vi "Accel Interpret.vi"(1 "LSB":u8, 2 "MSB":u8) -> (0 "Value":i16)   [LabVIEW 2010]
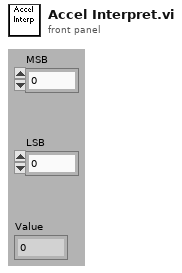
[diagram p1: front panel]
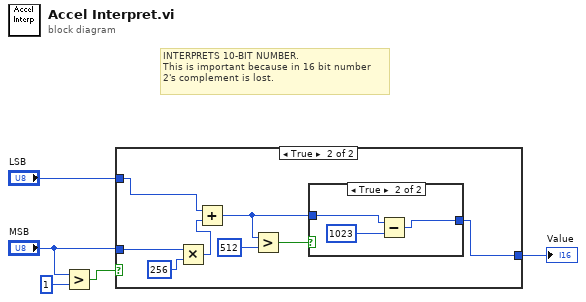
[diagram p0: block diagram]
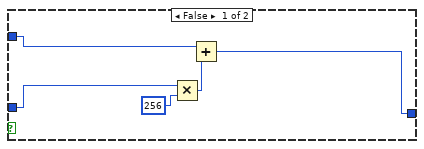
[diagram p2: hidden frame]
diagram:
  # "INTERPRETS 10-BIT NUMBER.\nThis is important because in 16 bit number\n2's complement is lost."
  n1 = Greater?(x="MSB", y=i16 1) -> (0:w4:bool)
  n2 = case shown="True" w4 {
    tunnel: "MSB" -> [w7 w13]
    tunnel: "LSB" -> [w8 w14]
    tunnel: [w6 w15] -> w5
    frame False {
      n3 = Multiply(x=w7, y=u16 256) -> (x*y=w9:u16)
      n4 = Add(x=w8, y=w9) -> (x+y=w6:u16)
    }
    frame True {
      n5 = Multiply(x=w13, y=i16 256) -> (x*y=w12:i16)
      n6 = Add(x=w14, y=w12) -> (x+y=w11:i16)
      n7 = Greater?(x=w11, y=i16 512) -> (0:w17:bool)
      n8 = case shown="True" w17 {
        tunnel: w11 -> [w19 w21]
        tunnel: [w19 w20] -> w15
        frame False {
        }
        frame True {
          n9 = Subtract(x=w21, y=i16 1023) -> (x-y=w20:i16)
        }
      }
    }
  }
  "Value" <- w5
